vi "Listen To Msg.vi"(7 "Actor in":refnum<class "Actor.lvclass">, 10 "Msg":refnum<class "Msg.lvclass">) -> (0 "Error out":errorcluster, 5 "Actor out":refnum<class "Actor.lvclass">)   [LabVIEW 2020, in "jettl.lvlib"]
uses:
  jettl.lvlib
  Actor/Actor.lvclass
  Msg/Msg.lvclass
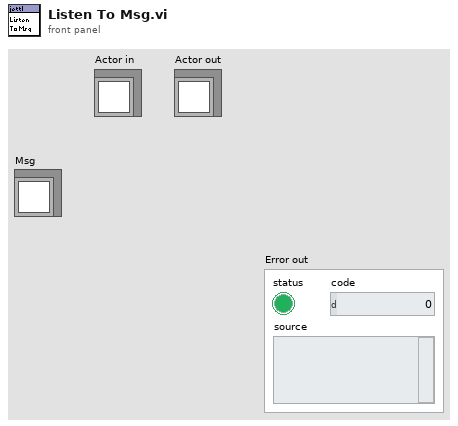
[diagram p1: front panel]
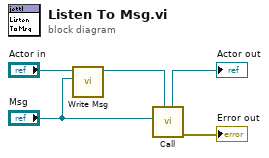
[diagram p0: block diagram]
diagram:
  n1 = call-dynamic "Write Msg.vi"("Msg"="Msg", "Actor in"="Actor in") -> ("Actor out"=w2:refnum<class "Actor.lvclass">)  [unwired: 9 in]
  n2 = call "Call.vi"("Actor in"=w2, "Msg"="Msg") -> ("Error out"=→"Error out":errorcluster, "Actor out"=→"Actor out":refnum<class "Actor.lvclass">)  [unwired: 7 in, 1 out]
